vi "Main.vi"(0 "VI Reference In":refnum<vi>, 7 "Control Name":string, 11 "error In":errorcluster) -> (4 "VI Reference Out":refnum<vi>, 15 "error out":errorcluster)   [LabVIEW 2016]
uses:
  main/apis/Setup/GetControlRef/GetControlRef.lvlib
  main/Drona.lvlib
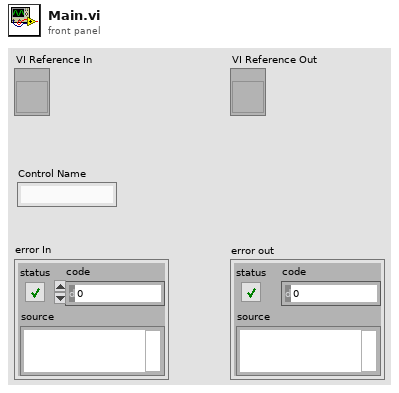
[diagram p1: front panel]
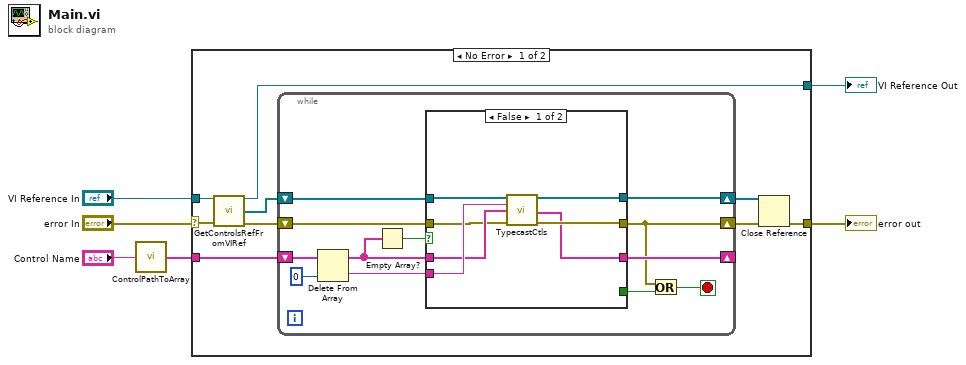
[diagram p0: block diagram]
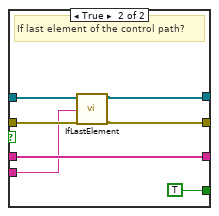
[diagram p2: hidden frame]
diagram:
  n1 = call "ControlPathToArray.vi"("Control Name"="Control Name") -> ("Control Path"=w2:string[])  [unwired: 1 in]
  n2 = case shown="No Error" "error In" {
    selector: "error In" -> [w9 w43]
    tunnel: w2 -> [w14 _]
    tunnel: [w8 w43] -> w6
    tunnel: "VI Reference In" -> [w10 w42]
    tunnel: [w7 w42] -> w3
    frame No Error {
      n3 = call "GetControlsRefFromVIRef.vi"("VI Reference In"=w10, "Error In"=w9) -> ("VI Reference Out"=w7:refnum<vi>, "Controls[]"=w13:refnum<vi>[], "Error Out"=w11:errorcluster)  [unwired: 11 in]
      n4 = while {
        shift-right: [w17] -> w15
        shift-left: w11 -> [w25]
        shift-right: [w22] -> w12
        shift-left: w13 -> [w23]
        shift-right: [w21] -> _
        shift-left: w14 -> [w24]
        stop <- w16 stop-if-true
        n5 = Delete From Array(array=w24, index=0) -> (deleted portion=w26:string, array with subset deleted=w20:string[])  [unwired: 1 in]
        n6 = Empty Array?(array=w20) -> (empty?=w27:bool)
        n7 = case shown="False" w27 {
          tunnel: w23 -> [w32 w37]
          tunnel: w26 -> [w34 w38]
          tunnel: w25 -> [w31 w39]
          tunnel: [w29 w35] -> w17
          tunnel: [w30 w36] -> w22
          tunnel: [_ TRUE] -> w18
          tunnel: w20 -> [w33 w40]
          tunnel: [w28 w40] -> w21
          frame False {
            n8 = call "TypecastCtls.vi"("Controls[]"=w32, "Control Name"=w34, "Control Path In"=w33, "error In"=w31) -> ("Sub Controls[]"=w30:refnum<vi>[], "Control Path Out"=w28:string[], "error out"=w29:errorcluster)  [unwired: 9 in]
          }
          frame True {
            # "If last element of the control path?"
            n9 = call "IfLastElement.vi"("Controls[]"=w37, "Control Path"=w38, "error In"=w39) -> ("Remaining Controls[]"=w36:refnum<vi>[], "error out"=w35:errorcluster)  [unwired: 11 in]
          }
        }
        n10 = Or(x=w17, y=w18) -> (x .or. y?=w16:bool)
      }
      n11 = Close Reference(reference=w12, error in (no error)=w15) -> (error out=w8:errorcluster)
    }
    frame Error {
    }
  }
  "error out" <- w6
  "VI Reference Out" <- w3
